vi "User Interface.vi"(8 "error in (no error)":errorcluster, 11 "User Interface in":refnum<class "User Interface.lvclass">) -> (0 "error out":errorcluster, 3 "User Interface out":refnum<class "User Interface.lvclass">)   [LabVIEW 2019, in "DSF Core.lvlib" / "Core Transfer User Interface.lvclass"]
uses:
  Core Transfer User Interface.lvclass
  User Interface.lvclass
  Configuration/Core/Transfer/Transfer Configuration.lvclass
  C:/Dev/GitHub/niveristand-data-sharing-framework-custom-device/Core/Classes/Configuration/Configuration.lvclass
  Configuration/Core/Transfer/Transfer Configuration.lvclass/Transfer Configuration.ctl
  Configuration/Configuration.lvclass
panel:
  in  "Name":string
  out "Data Version":string
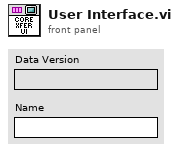
[diagram p1: front panel]
types:
  T1 = typedef "DSF Core.lvlib/Transfer Configuration.lvclass/Core Transfer Configuration.ctl" = cluster{"name":string}
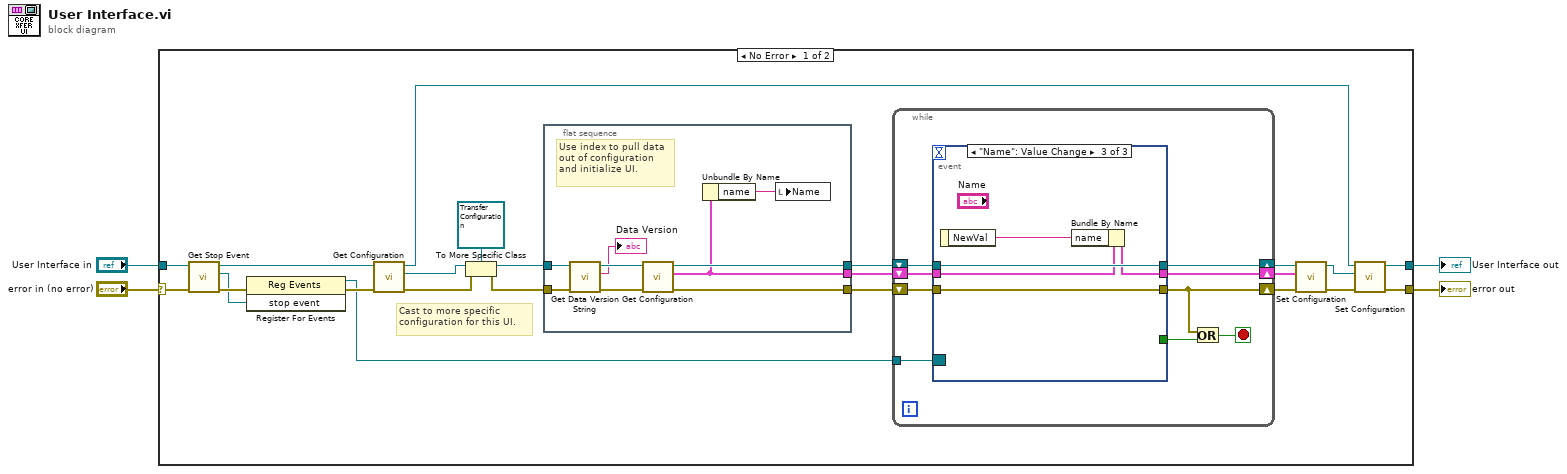
[diagram p0: block diagram]
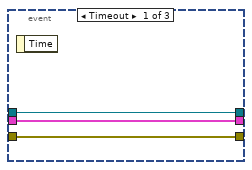
[diagram p2: hidden frame]
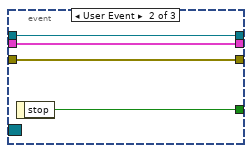
[diagram p3: hidden frame]
diagram:
  n1 = case shown="No Error" "error in (no error)" {
    selector: "error in (no error)" -> [w21 w59]
    tunnel: [w14 w59] -> w4
    tunnel: "User Interface in" -> [w20 w58]
    tunnel: [w13 w58] -> w1
    frame No Error {
      # "Cast to more specific configuration for this UI."
      n2 = call "Get Stop Event.vi"("error in (no error)"=w21, "User Interface in"=w20) -> ("error out"=w19:errorcluster, "stop event"=w18:refnum<user-event>, "User Interface out"=w22:refnum<class "User Interface.lvclass">)  [unwired: 7 in]
      n3 = register-events(error in=w19, w18) -> (reference out=w11:refnum<event-registration>, error out=w17:errorcluster)  [unwired: 1 in]
      n4 = call "Get Configuration.vi"("error in (no error)"=w17, "User Interface in"=w22) -> ("error out"=w16:errorcluster, "configuration"=w15:refnum<class "Configuration.lvclass">, "User Interface out"=w12:refnum<class "User Interface.lvclass">)  [unwired: 7 in]
      n5 = To More Specific Class(target class=refnum<class "Transfer Configuration.lvclass"> refnum ("DSF Core.lvlib:Transfer Configuration.lvclass"), reference=w15, error in=w16) -> (specific class reference=w27:refnum<class "Transfer Configuration.lvclass">, error out=w24:errorcluster)
      n6 = flat-sequence {
        tunnel: [w30] -> w25
        tunnel: w24 -> [w36]
        tunnel: w27 -> [w35]
        tunnel: [w31] -> w26
        tunnel: [w29] -> w23
        frame #0 {
          # "Use index to pull data out of configuration and initialize UI."
          n7 = call "Get Data Version String.vi"("error in (no error)"=w36, "Configuration in"=w35) -> ("error out"=w33:errorcluster, "data version"=→"Data Version":string, "Configuration out"=w32:refnum<class "Transfer Configuration.lvclass">)  [unwired: 7 in]
          n8 = call "Get Configuration.vi"("error in (no error)"=w33, "Core Transfers Configuration in"=w32) -> ("error out"=w30:errorcluster, "configuration"=w29:T1, "Core Transfers Configuration out"=w31:refnum<class "Transfer Configuration.lvclass">)  [unwired: 7 in]
          n9 = Unbundle By Name(w29) -> ("name"=w34:string)
          n10 = local write "Name"(w34) -> ()
        }
      }
      n11 = while {
        tunnel: w11 -> [w45]
        shift-right: [w43] -> w8
        shift-left: w25 -> [w44]
        shift-right: [w39] -> w9
        shift-left: w26 -> [w40]
        shift-right: [w37] -> w5
        shift-left: w23 -> [w38]
        stop <- w42 stop-if-true
        n12 = event shown="[2] \"Name\": Value Change" {
          selector: w45 -> [_ _ _]
          dyn-events: _ -> [_ _ _]
          timeout: _ -> [_ _ _]
          tunnel: [_ w50 _] -> w41
          tunnel: w44 -> [w48 w52 w57]
          tunnel: [w48 w52 w57] -> w43
          tunnel: w40 -> [w47 w51 w56]
          tunnel: [w47 w51 w56] -> w39
          tunnel: w38 -> [w46 w49 w53]
          tunnel: [w46 w49 w55] -> w37
          event Timeout {
            n13 = event-data() -> ()  [unwired: 1 in, 1 out]
          }
          event User Event {
            n14 = event-data() -> ("stop"=w50:bool)  [unwired: 1 in]
          }
          event "Name": Value Change {
            n15 = event-data() -> ("NewVal"=w54:string)  [unwired: 1 in]
            n16 = Bundle By Name(cluster=w53, "name"=w54) -> (w55:T1)
          }
        }
        n17 = Or(x=w43, y=w41) -> (x .or. y?=w42:bool)
      }
      n18 = call "Set Configuration.vi"("error in (no error)"=w8, "configuration"=w5, "Core Transfers Configuration in"=w9) -> ("error out"=w7:errorcluster, "Core Transfers Configuration out"=w6:refnum<class "Transfer Configuration.lvclass">)  [unwired: 7 in]
      n19 = call "Set Configuration.vi"("error in (no error)"=w7, "configuration"=w6, "User Interface in"=w12) -> ("error out"=w14:errorcluster, "User Interface out"=w13:refnum<class "User Interface.lvclass">)  [unwired: 7 in]
    }
    frame Error {
    }
  }
  "error out" <- w4
  "User Interface out" <- w1
